vi "DataLog[1072].vi"() -> ()   [LabVIEW 2018]
panel:
  in  "Log Rate (Sec)":fxp<+,32,32>
  out "PATH":path
  out "error out":errorcluster
  out "Elapsed Time (s)":dbl
  in  "File Name":string
  out "Sine Value":dbl
  in  "Amplitude":dbl=100.0
  in  "Frequency":dbl=10.1
  in  "Record Data":bool
  in  "Slow Sine":dbl(slide) scale=0.0..1.0
  out "Waveform Graph":dynamicdata(graph)
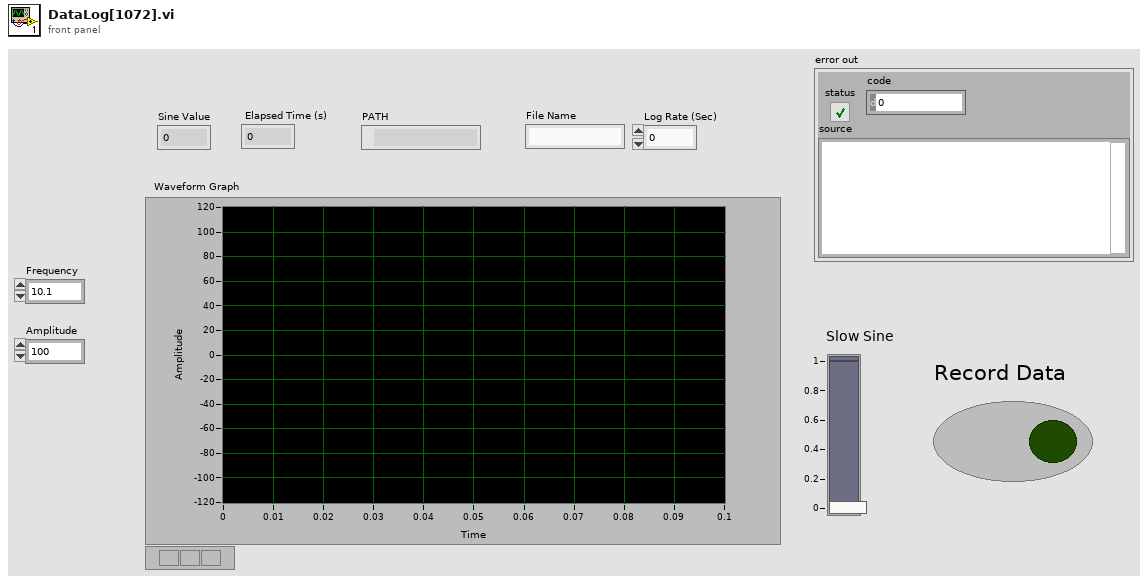
[diagram p1: front panel]
types:
  T1 = enum16{"open", "replace", "create", "open or create", "replace or create", "replace or create with confirmation"}
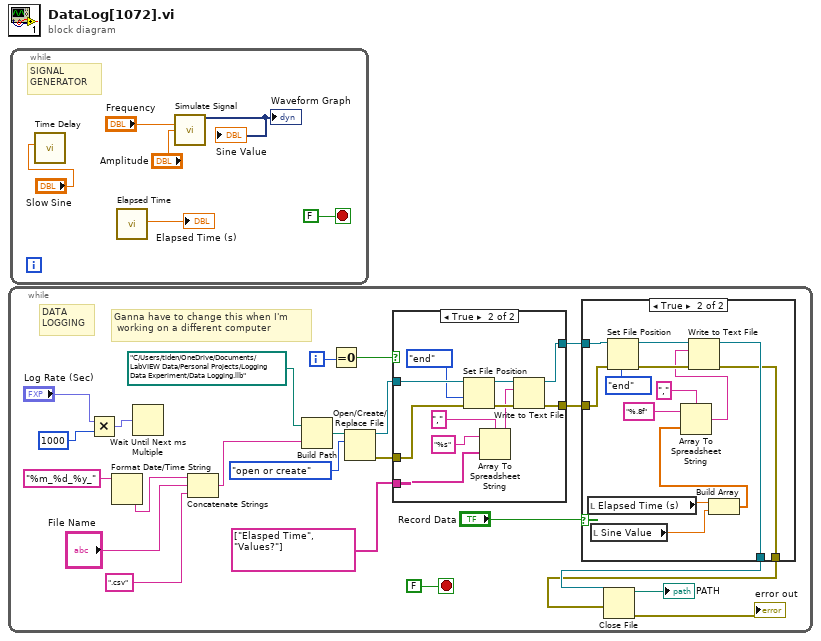
[diagram p0: block diagram]
diagram:
  n1 = while {
    i -> [w14]
    stop <- FALSE stop-if-true
    # "DATA\nLOGGING"
    # "Ganna have to change this when I'm\n working on a different computer"
    n2 = Multiply(x="Log Rate (Sec)", y=1000) -> (x*y=w3:fxp<+/-,64,64>)
    n3 = Format Date/Time String(time format string (%c)="%m_%d_%y_") -> (date/time string=w22:string)  [unwired: 2 in]
    n4 = Wait Until Next ms Multiple(millisecond multiple=w3) -> ()  [unwired: 1 out]
    n5 = Concatenate Strings(w22, "File Name", ".csv" ("string")) -> (w21:string)
    n6 = Build Path(base path=path "C:/Users/tiden/OneDrive/Documents/LabVIEW Data/Personal Projects/Logging Data Experiment/Data Logging.llb", name or relative path=w21) -> (appended path=w19:path)
    n7 = Equal To 0?(x=w14) -> (x = 0?=w13:bool)
    n8 = Open/Create/Replace File(file path (use dialog)=w19, operation (0:open)=T1."open or create") -> (refnum out=w23:refnum<file>, error out=w24:errorcluster)  [unwired: 4 in, 1 out]
    n9 = case shown="True" w13 {
      tunnel: w23 -> [w40 w51]
      tunnel: w24 -> [w41 w49]
      tunnel: string[] ["Elasped Time", "Values?"] ("string array") -> [_ w44]
      tunnel: [w40 w43] -> w9
      tunnel: [w41 w42] -> w8
      frame False {
      }
      frame True {
        n10 = Set File Position(refnum=w51, from (0:start)=enum16{"start", "end", "current"}."end", error in=w49) -> (refnum out=w52:refnum<file>, error out=w48:errorcluster)  [unwired: 1 in]
        n11 = Array To Spreadsheet String(delimiter (Tab)=",", array=w44, 3:"%s" ("format string")) -> (spreadsheet string=w47:string)
        n12 = Write to Text File(file (use dialog)=w52, text=w47, error in=w48) -> (refnum out=w43:refnum<file>, error out=w42:errorcluster)  [unwired: 1 in, 1 out]
      }
    }
    n13 = case shown="True" "Record Data" {
      tunnel: w9 -> [w25 w39]
      tunnel: w8 -> [w26 w38]
      tunnel: [w25 w28] -> w7
      tunnel: [w26 w27] -> w6
      frame False {
      }
      frame True {
        n14 = local read "Elapsed Time (s)"() -> (w34:dbl)
        n15 = local read "Sine Value"() -> (w33:dbl)
        n16 = Set File Position(refnum=w39, from (0:start)=enum16{"start", "end", "current"}."end", error in=w38) -> (refnum out=w37:refnum<file>, error out=w36:errorcluster)  [unwired: 1 in]
        n17 = Build Array(w34, w33) -> (w29:dbl[])
        n18 = Array To Spreadsheet String(delimiter (Tab)=",", array=w29, 3:"%.8f" ("format string")) -> (spreadsheet string=w32:string)
        n19 = Write to Text File(file (use dialog)=w37, text=w32, error in=w36) -> (refnum out=w28:refnum<file>, error out=w27:errorcluster)  [unwired: 1 in, 1 out]
      }
    }
    n20 = Close File(refnum=w7, error in=w6) -> (path=→"PATH":path, error out=→"error out":errorcluster)
  }
  n21 = while {
    stop <- FALSE stop-if-true
    # "SIGNAL \nGENERATOR"
    n22 = call "Time Delay"("Delay Time (s)"="Slow Sine") -> ()  [unwired: 10 in, 1 out]
    n23 = call "Elapsed Time"() -> ("Elapsed Time (s)"=→"Elapsed Time (s)":dbl)  [unwired: 12 in, 7 out]
    n24 = call "Simulate Signal"("Frequency"="Frequency", "Amplitude"="Amplitude") -> ("Sine with Uniform Noise"=→"Waveform Graph" →"Sine Value":dynamicdata)  [unwired: 12 in, 1 out]
  }
